vi "FindROIstring.vi"(10 "ROI":string="r=[0,0,320,240]", 11 "ROI":T1) -> (2 "Cluster":T1, 3 "String":string)   [LabVIEW 2022 SP3]
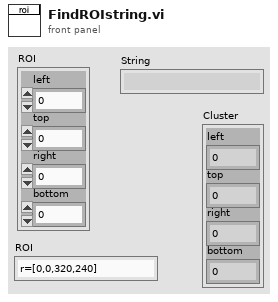
[diagram p1: front panel]
types:
  T1 = cluster{"left":i32, "top":i32, "right":i32, "bottom":i32}
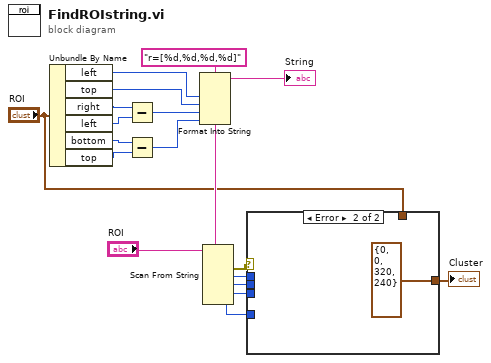
[diagram p0: block diagram]
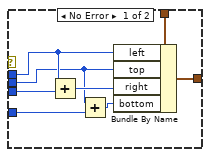
[diagram p2: hidden frame]
diagram:
  w9 = "r=[%d,%d,%d,%d]" ("format string")
  n1 = Unbundle By Name("ROI") -> ("left"=w15:i32, "top"=w17:i32, "right"=w10:i32, "left"=w11:i32, "bottom"=w12:i32, "top"=w16:i32)
  n2 = Subtract(x=w10, y=w11) -> (x-y=w13:i32)
  n3 = Subtract(x=w12, y=w16) -> (x-y=w14:i32)
  n4 = Format Into String(format string=w9, w15, w17, w13, w14) -> (resulting string=→"String":string)  [unwired: 2 in, 1 out]
  n5 = Scan From String(format string=w9, input string="ROI") -> (error out=w1:errorcluster, output 1=w6:i32, output 2=w4:i32, output 3=w5:i32, output 4=w3:i32)  [unwired: 6 in, 2 out]
  n6 = case shown="Error" w1 {
    tunnel: "ROI" -> [w26 _]
    tunnel: w6 -> [w25 _]
    tunnel: w5 -> [w24 _]
    tunnel: w4 -> [w22 _]
    tunnel: w3 -> [w21 _]
    tunnel: [w19 T1 {"left"=0, "top"=0, "right"=320, "bottom"=240} ("ROI")] -> w2
    frame No Error {
      n7 = Add(x=w24, y=w25) -> (x+y=w23:i32)
      n8 = Add(x=w22, y=w21) -> (x+y=w20:i32)
      n9 = Bundle By Name(cluster=w26, "left"=w25, "top"=w22, "right"=w23, "bottom"=w20) -> (w19:T1)
    }
    frame Error {
    }
  }
  "Cluster" <- w2
